vi "Stop Core.vi"(10 "final error code":i32, 11 "WebSocket Connection in":refnum<class "WebSocket Connection.lvclass">) -> (3 "WebSocket Connection out":refnum<class "WebSocket Connection.lvclass">)   [LabVIEW 2016, in "WebSocket Actors.lvlib" / "WebSocket Connection.lvclass"]
doc: "(<B>Filename</B>: Actor Framework.lvlib:Actor.lvclass:Stop Core.vi)\n\nDefines what the actor does before it stops. Use the <B>final error code</B> input to determine whether the actor shut down in response to an error.\n\nBy default, this method does nothing. A descendant class may override it to define behavior, such as shutting down any processes the actor initiated in its override of the Actor Core method."
uses:
  WebSocket Connection.lvclass
  Abstract Messages/WebSocket Connection Handler Msg/typedefs/Message Data.ctl
  <vilib>/ActorFramework/Message Enqueuer/Message Enqueuer.lvclass
  Websockets/Data Format.ctl
  WebSocket Connection.lvclass/WebSocket Connection.ctl
  Abstract Messages/WebSocket Connection Handler Msg/properties/Connection Event.ctl
  Websockets/StatusCode.ctl
  Abstract Messages/WebSocket Connection Handler Msg/WebSocket Connection Handler Msg.lvclass/WebSocket Connection Handler Msg.ctl
  <vilib>/ActorFramework/Message Enqueuer/Message Enqueuer.lvclass/Message Enqueuer.ctl
  <vilib>/ActorFramework/Message Enqueuer/Enqueue.vi
  Abstract Messages/WebSocket Connection Handler Msg/WebSocket Connection Handler Msg.lvclass
  C:/Program Files (x86)/National Instruments/LabVIEW 2016/vi.lib/ActorFramework/Message/Message.lvclass
  <vilib>/ActorFramework/Message Priority Queue/Priority Enqueue.vi
  <vilib>/MGI/Monitored Actor/Monitored Actor/Monitored Actor/Monitored Actor.lvclass
  Websockets/WebSockets.lvlib
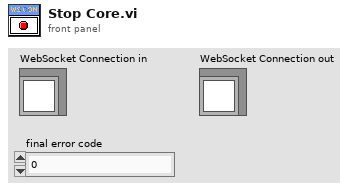
[diagram p1: front panel]
types:
  T1 = typedef "WebSocket Actors.lvlib/WebSocket Connection Handler Msg.lvclass/Message Data.ctl" = cluster{"Data":string, "Peer ID":string, "Connection Enqueuer":refnum<class "Message Enqueuer.lvclass">, "Data Format":T2}
  T2 = typedef "WebSockets.lvlib/Data Format.ctl" = enum16{"Text", "Binary"}
  T3 = typedef "WebSocket Actors.lvlib/WebSocket Connection.lvclass/Connection Status.ctl" = enum16{"Open", "Closed by Self", "Closed by Peer", "Dropped"}
  T4 = typedef "WebSocket Actors.lvlib/WebSocket Connection Handler Msg.lvclass/Connection Event.ctl" = enum16{"On Connect", "On Message", "On Close", "On Drop"}
  T5 = typedef "WebSockets.lvlib/StatusCode.ctl" = u16
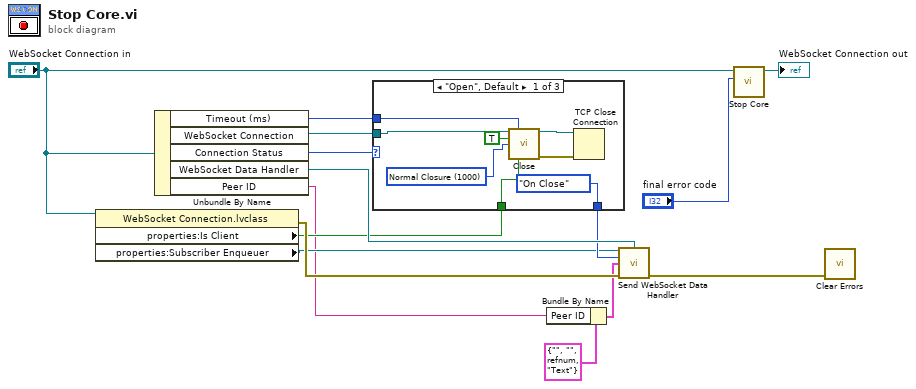
[diagram p0: block diagram]
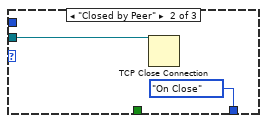
[diagram p2: hidden frame]
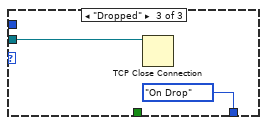
[diagram p3: hidden frame]
diagram:
  n1 = property class="WebSocket Connection.lvclass"(reference="WebSocket Connection in") -> (error out=w7:errorcluster, "properties:Is Client"=w5:bool, "properties:Subscriber Enqueuer"=w6:refnum<class "Message Enqueuer.lvclass">)  [unwired: 1 in, 1 out]
  n2 = Unbundle By Name("WebSocket Connection in") -> ("Timeout (ms)"=w1:i32, "WebSocket Connection"=w13:refnum<k5>, "Connection Status"=w12:T3, "WebSocket Data Handler"=w11:refnum<class "WebSocket Connection Handler Msg.lvclass">, "Peer ID"=w3:string)
  n3 = case shown="\"Open\", Default" w12 {
    tunnel: w13 -> [w23 w25 w27]
    tunnel: [Connection_Event."On Close" ("Connection Event") Connection_Event."On Close" ("Connection Event") Connection_Event."On Drop" ("Connection Event")] -> w9
    tunnel: w5 -> [w17 _ _]
    tunnel: w1 -> [w16 _ _]
    frame "Open", Default {
      w18 = T5 1000 items=["Normal Closure"=1000, "Going Away"=1001, "Protocol Error"=1002, "Wrong Data Type"=1003, "Reserved 1004"=1004, "Reserved 1005"=1005, "Reserved 1006"=1006, "Non Consistent Data Type"=1007, "Policy Violation"=1008, "Message Too Big"=1009, "Extensions Negotiation Error"=1010, "Unexpected Condition"=1011, "Reserved 1015"=1015] ("Status Code")
      n4 = call "Close.vi"("WebSocket Connection in"=w23, "timeout ms (5000)"=w16, "Send Reason (F)"=TRUE, "Status Code"=w18, "Mask payload?"=w17) -> ("WebSocket Connection in"=w21:refnum<k5>, "error out"=w22:errorcluster)  [unwired: 9 in]
      n5 = TCP Close Connection(connection ID=w21, error in (no error)=w22) -> ()  [unwired: 1 in, 2 out]
    }
    frame "Closed by Peer" {
      n6 = TCP Close Connection(connection ID=w25) -> ()  [unwired: 2 in, 2 out]
    }
    frame "Dropped" {
      n7 = TCP Close Connection(connection ID=w27) -> ()  [unwired: 2 in, 2 out]
    }
  }
  n8 = Bundle By Name(cluster=T1 {"Data"="", "Peer ID"="", "Connection Enqueuer"=refnum, "Data Format"=enum."Text"} ("Connection Message Data"), "Peer ID"=w3) -> (w2:T1)
  n9 = call "Send WebSocket Data Handler.vi"("Message Enqueuer"=w6, "Message Type"=w11, "Connection Event"=w9, "Connection Message Data"=w2, "error in (no error)"=w7) -> ("error out"=w10:errorcluster)  [unwired: 9 in, 1 out]
  n10 = call-parent "Stop Core.vi"("final error code"="final error code", "Monitored Actor in"="WebSocket Connection in") -> ("Monitored Actor out"=→"WebSocket Connection out":refnum<class "WebSocket Connection.lvclass">)  [unwired: 9 in]
  n11 = call <vilib>:"Clear Errors.vi"("error in (no error)"=w10) -> ()  [unwired: 5 in, 2 out]
